vi "AutoMatch(P4).vi"() -> ()   [LabVIEW 2019]
panel:
  out "# of Iterations":i32
  out "Current Number":dbl format="%#.0f"
  in  "Match a Number":dbl min=0.0 max=1000.0 step=1.0 format="%#.0f"
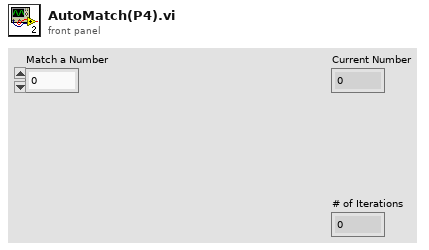
[diagram p1: front panel]
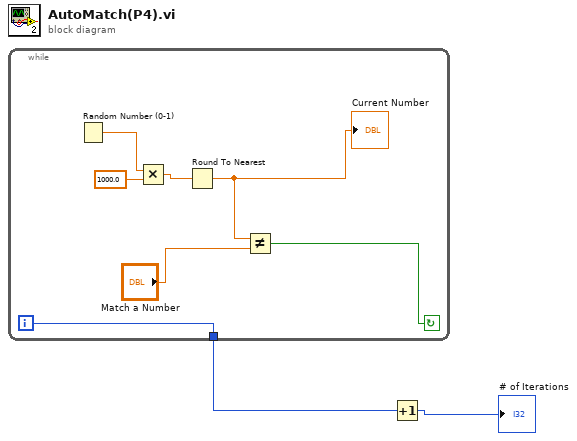
[diagram p0: block diagram]
diagram:
  n1 = while {
    tunnel: [w3] -> w1
    i -> [w3]
    stop <- w6 continue-if-true
    n2 = Random Number (0-1)() -> (number: 0 to 1=w9:dbl)
    n3 = Multiply(x=w9, y=1000.0) -> (x*y=w7:dbl)
    n4 = Round To Nearest(number=w7) -> (nearest integer value=w5:dbl)
    "Current Number" <- w5
    n5 = Not Equal?(x=w5, y="Match a Number") -> (x != y?=w6:bool)
  }
  n6 = Increment(x=w1) -> (x+1=→"# of Iterations":i32)
